vi "RFSG Configure Trigger.vi"(8 "error in (no error)":errorcluster, 11 "RFSG Reference In":refnum<k15>) -> (0 "error out":errorcluster, 3 "RFSG Reference Out":refnum<k15>)   [LabVIEW 2021]
uses:
  <instrlib>/niRFSG/niRFSG.llb/niRFSG Signal Names.ctl
  <instrlib>/niRFSG/niRFSG.llb/niRFSG Signal Identifiers.ctl
  <instrlib>/niRFSG/niRFSG.llb/niRFSG Exported Signal Destinations.ctl
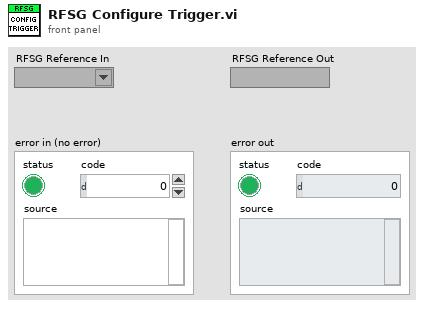
[diagram p1: front panel]
types:
  T1 = typedef "niRFSG Exported Signal Destinations.ctl" = string
  T2 = typedef "niRFSG Signal Identifiers.ctl" = string
  T3 = typedef "niRFSG Signal Names.ctl" = i32
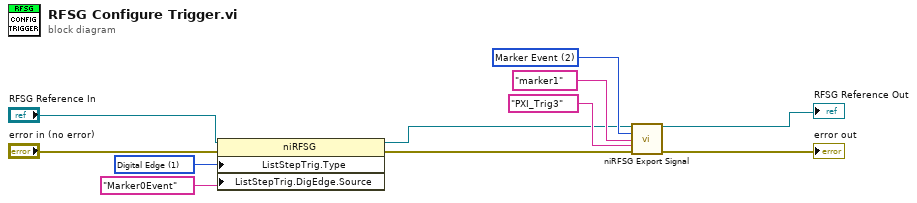
[diagram p0: block diagram]
diagram:
  w8 = T3 2 items=["Start Trigger", "Script Trigger", "Marker Event", "Ref Clock", "Started Event", "Done Event", "Configuration List Step Trigger", "Configuration Settled Event"] ("signal")
  w3 = 1 items=["None", "Digital Edge", "Software"] ("Triggers:Configuration List Step:Type")
  n1 = property class="niRFSG"(reference="RFSG Reference In", error in="error in (no error)", "ListStepTrig.Type"=w3, "ListStepTrig.DigEdge.Source"="Marker0Event" ("Triggers:Configuration List Step:Digital Edge:Source")) -> (reference out=w5:refnum<k15>, error out=w6:errorcluster)
  n2 = call <instrlib>:"niRFSG Export Signal.vi"("instrument handle"=w5, "signal"=w8, "signal identifier"=T2 "marker1", "output terminal"=T1 "PXI_Trig3", "error in"=w6) -> ("instrument handle out"=→"RFSG Reference Out":refnum<k15>, "error out"=→"error out":errorcluster)  [unwired: 9 in]
